vi "Get State.vi"(8 "error in (no error)":errorcluster, 11 "Worker in":refnum<class "Worker.lvclass">) -> (0 "error out":errorcluster, 1 "Result ready":bool, 2 "Armed":bool, 3 "Worker out":refnum<class "Worker.lvclass">, 4 "Check again":bool)   [LabVIEW 2018, in "Worker.lvclass"]
uses:
  Worker.lvclass
  Worker.lvclass/Worker.ctl
  Template Module/Read State.vi
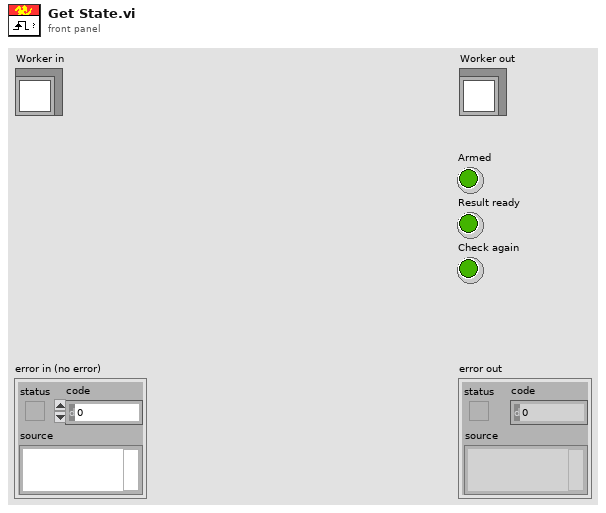
[diagram p1: front panel]
types:
  T1 = typedef "Worker State.ctl" = enum16{"Idle", "Starting", "Working", "Stopping"}
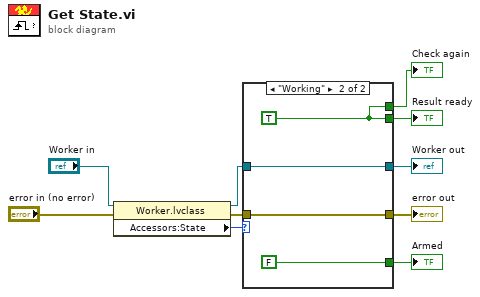
[diagram p0: block diagram]
diagram:
  n1 = property class="Worker.lvclass"(reference="Worker in", error in="error in (no error)") -> (reference out=w7:refnum<class "Worker.lvclass">, error out=w6:errorcluster, "Accessors:State"=w4:T1)
  n2 = case shown="\"Working\"" w4 {
    tunnel: [w11 w15] -> w10
    tunnel: [w12 w16] -> w9
    tunnel: w7 -> [w12 w16]
    tunnel: w6 -> [w11 w15]
    tunnel: [_ FALSE ("Armed")] -> w3
    tunnel: [_ w13] -> w2
    tunnel: [_ w13] -> w1
    frame "Idle", Default {
    }
    frame "Working" {
      w13 = TRUE ("Data ready")
    }
  }
  "error out" <- w10
  "Worker out" <- w9
  "Armed" <- w3
  "Result ready" <- w2
  "Check again" <- w1
